vi "MATLAB script node - Fractal.vi"() -> ()   [LabVIEW 2023]
doc: "Demonstrates how to use the MATLAB script node. The m-file script is used to calculate the data and the resulting fractal is displayed on the front panel. The MathWorks, Inc. MATLAB (R) Application Software version 5.0 or later must be installed and properly licensed in order to run this VI."
panel:
  out "Calculation Time (s)":dbl
  out "Fractal Plot":dbl[][](graph)
  # "Overview: Generates a fractal using the MATLAB script node and plots the result.\nRequirements: LabVIEW Full Development System, The MathWorks, Inc. MATLAB (R) Application Software version 5.0 or later\nInstructions:\nRun the VI."
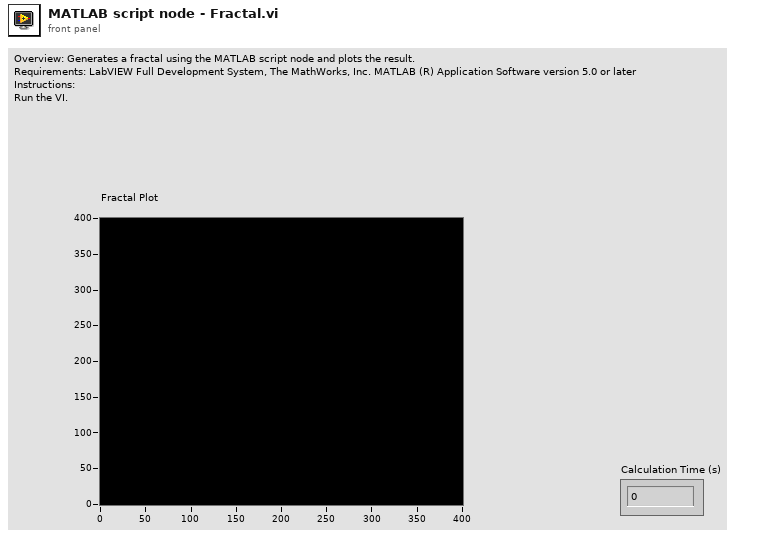
[diagram p1: front panel]
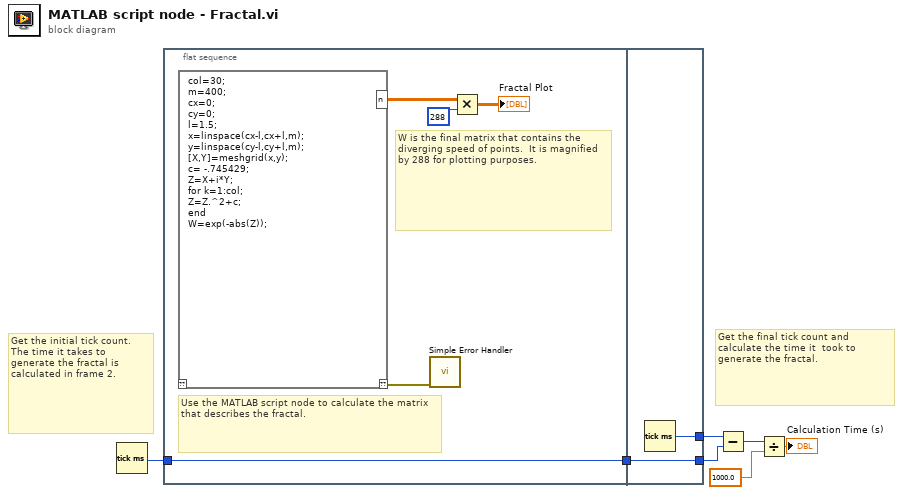
[diagram p0: block diagram]
diagram:
  # "Get the final tick count and calculate the time it  took to generate the fractal."
  # "Get the initial tick count.  The time it takes to generate the fractal is calculated in frame 2."
  n1 = Tick Count (ms)() -> (millisecond timer value=w6:u32)
  n2 = flat-sequence {
    tunnel: [w10] -> w7
    tunnel: w6 -> [w10]
    tunnel: w7 -> [w13]
    tunnel: [w14] -> w3
    tunnel: [w13] -> w2
    frame #0 {
      # "Use the MATLAB script node to calculate the matrix that describes the fractal."
      # "W is the final matrix that contains the diverging speed of points.  It is magnified by 288 for plotting purposes."
      n3 = script code="col=30;\nm=400;\ncx=0;\ncy=0;\nl=1.5;\nx=linspace(cx-l,cx+l,m);\ny=linspace(cy-l,cy+l,m);\n[X,Y]=meshgrid(x,y);\nc= -.745429;\nZ=X+i*Y;\nfor k=1:col;\nZ=Z.^2+c;\nend\nW=exp(-abs(Z));"() -> ("??"=w8:errorcluster, "n"=w9:dbl[][])  [unwired: 1 in]
      n4 = call <vilib>:"Simple Error Handler.vi"("error in (no error)"=w8) -> ()  [unwired: 4 in, 5 out]
      n5 = Multiply(x=w9, y=288) -> (x*y=→"Fractal Plot":dbl[][])
    }
    frame #1 {
      n6 = Tick Count (ms)() -> (millisecond timer value=w14:u32)
    }
  }
  n7 = Subtract(x=w3, y=w2) -> (x-y=w4:u32)
  n8 = Divide(x=w4, y=1000.0) -> (x/y=→"Calculation Time (s)":dbl)
